vi "T-Flip-Flop.vi"(8 "Starting Value":bool, 11 "Flip":bool) -> (3 "Value":bool)   [LabVIEW 2018]
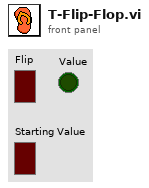
[diagram p1: front panel]
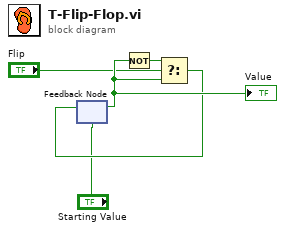
[diagram p0: block diagram]
diagram:
  n1 = feedback #1("Starting Value") -> (w4:bool)
  "Value" <- w4
  n2 = Not(x=w4) -> (.not. x?=w5:bool)
  n3 = Select(t=w5, s="Flip", f=w4) -> (s? t:f=w3:bool)
  n4 = feedback-in #1(w3) -> ()
